vi "MQTT_PubComp_Read.vi"(8 "error in (no error)":errorcluster, 11 "SSL_Connection":T1) -> (0 "error out":errorcluster, 2 "Message ID":u16=10 format="%x", 3 "SSL_Connection":T1)   [LabVIEW 2018, in "AWS_IoT.lvlib"]
doc: "© 2015 - daq.io, LLC - Peter Adelhardt"
uses:
  AWS_IoT.lvlib
  Controls/SSL_Connection.ctl
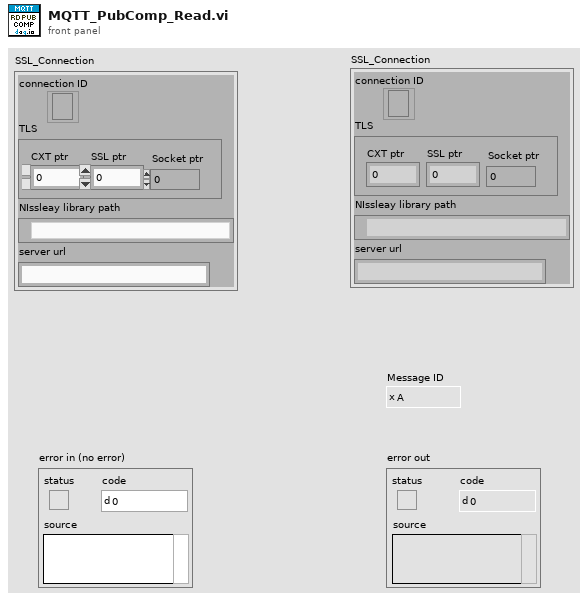
[diagram p1: front panel]
types:
  T1 = typedef "AWS_IoT.lvlib/SSL_Connection.ctl" = cluster{"connection ID":refnum<k5>, "TLS":cluster{"CXT ptr":i32, "SSL ptr":i32, "Socket ptr":i32}, "NIssleay library path":path, "server url":string}
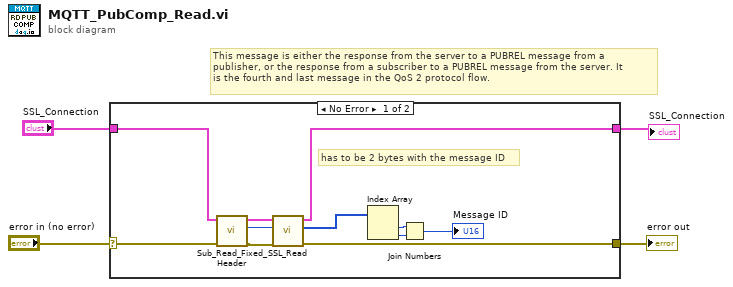
[diagram p0: block diagram]
diagram:
  # "This message is either the response from the server to a PUBREL message from a\npublisher, or the response from a subscriber to a PUBREL message from the server. It\nis the fourth and last message in the QoS 2 protocol flow."
  n1 = case shown="No Error" "error in (no error)" {
    selector: "error in (no error)" -> [w12 w17]
    tunnel: [w11 w17] -> w3
    tunnel: "SSL_Connection" -> [w6 w16]
    tunnel: [w5 w16] -> w1
    frame No Error {
      # "has to be 2 bytes with the message ID"
      n2 = call "Sub_Read_Fixed_Header.vi"("error in (no error)"=w12, "SSL_Connection"=w6) -> ("error out"=w9:errorcluster, "Remaining Length"=w10:u32, "SSL_Connection"=w7:T1)  [unwired: 3 in, 4 out]
      n3 = call "SSL_Read.vi"("error in (no error)"=w9, "bytes to read"=w10, "SSL_Connection"=w7) -> ("error out"=w11:errorcluster, "data out"=w8:u8[], "SSL_Connection"=w5:T1)  [unwired: 5 in, 1 out]
      n4 = Index Array(array=w8) -> (element #1=w14:u8, element #2=w15:u8)  [unwired: 2 in]
      n5 = Join Numbers(hi=w14, lo=w15) -> ((hi.lo)=→"Message ID":u16)
    }
    frame Error {
    }
  }
  "error out" <- w3
  "SSL_Connection" <- w1
